vi "Write Switch Channel.vi"(8 "error in (no error)":errorcluster, 10 "switch phys chan":tag, 11 "DAQmx Switch in":refnum<class "DAQmx Switch.lvclass">) -> (0 "error out":errorcluster, 3 "DAQmx Switch out":refnum<class "DAQmx Switch.lvclass">)   [LabVIEW 2020, in "DAQmx Switch.lvclass"]
uses:
  DAQmx Switch.lvclass
  DAQmx Switch.lvclass/DAQmx Switch.ctl
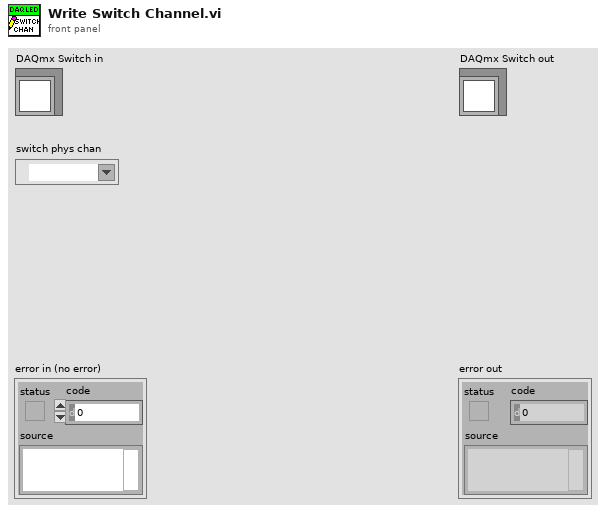
[diagram p1: front panel]
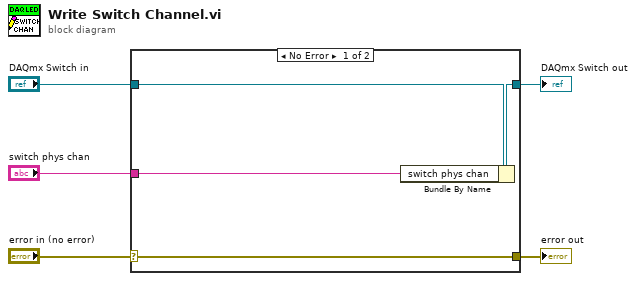
[diagram p0: block diagram]
diagram:
  n1 = case shown="No Error" "error in (no error)" {
    selector: "error in (no error)" -> [w9 w10]
    tunnel: [w9 w10] -> w4
    tunnel: [w7 w11] -> w2
    tunnel: "DAQmx Switch in" -> [w8 w11]
    tunnel: "switch phys chan" -> [w6 _]
    frame No Error {
      n2 = Bundle By Name(cluster=w8, "switch phys chan"=w6) -> (w7:refnum<class "DAQmx Switch.lvclass">)
    }
    frame Error {
    }
  }
  "error out" <- w4
  "DAQmx Switch out" <- w2
